vi "0254-initialization-reference.vi"(11 "0254-VISA":refnum<visa-resource-name>) -> (0 "error out":errorcluster, 2 "Executing Cmd":string, 3 "Execuiting Result":string)   [LabVIEW 2015]
uses:
  <vilib>/Instr/_visa.llb/VISA Configure Serial Port (Instr).vi
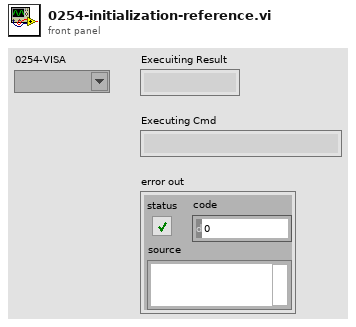
[diagram p1: front panel]
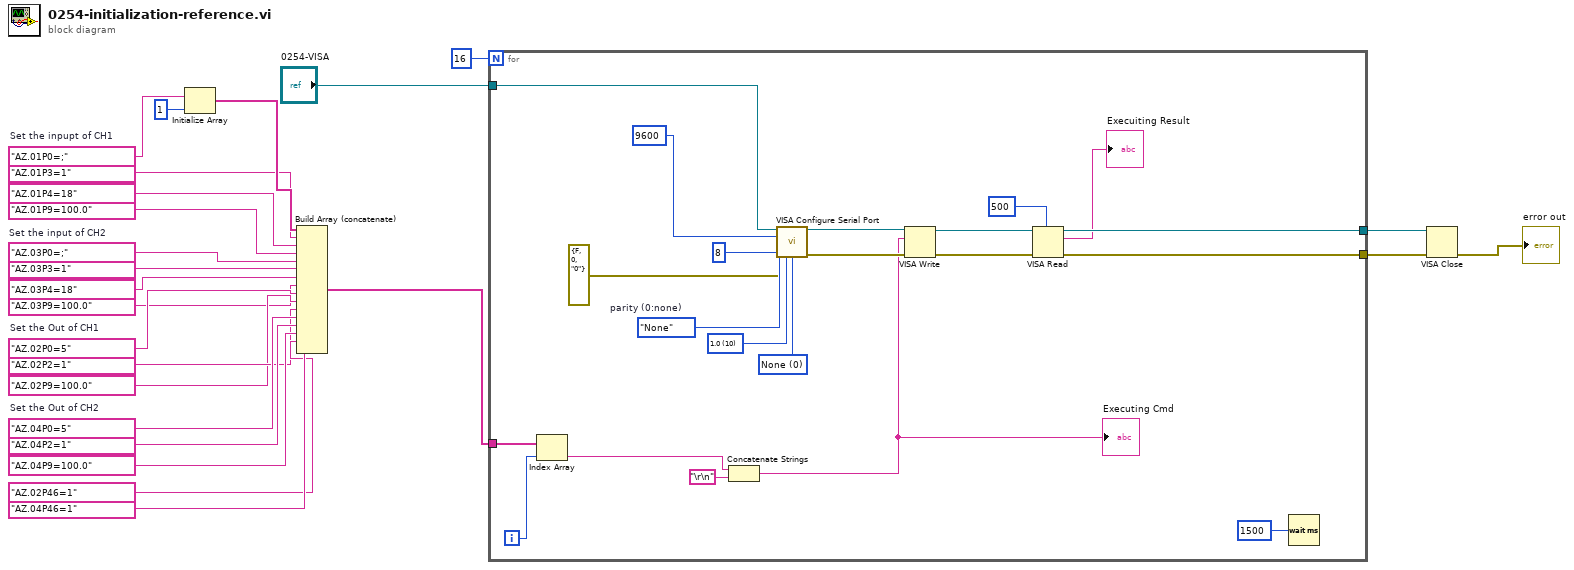
[diagram p0: block diagram]
diagram:
  w11 = "AZ.04P0=5"  # Set the Out of CH2
  w8 = "AZ.02P0=5"  # Set the Out of CH1
  w4 = "AZ.03P0=;"  # Set the input of CH2
  w18 = "AZ.01P0=;"  # Set the inpupt of CH1
  n1 = Initialize Array(w18, 1 ("dimension size")) -> (w20:string[])
  n2 = Build Array (concatenate)(w20, "AZ.01P3=1", "AZ.01P4=18", "AZ.01P9=100.0", w4, "AZ.03P3=1", "AZ.03P4=18", "AZ.03P9=100.0", w8, "AZ.02P9=100.0", "AZ.02P2=1", w11, "AZ.04P2=1", "AZ.04P9=100.0", "AZ.02P46=1", "AZ.04P46=1") -> (w21:string[])
  n3 = for {
    N: 16 -> [_]
    tunnel: [w29] -> w15
    tunnel: [w28] -> w16
    tunnel: "0254-VISA" -> [w27]
    tunnel: w21 -> [w26]
    i -> [w32]
    w37 = u16 0 items=["None", "XON/XOFF", "RTS/CTS", "XON/XOFF & RTS/CTS", "DTR/DSR", "XON/XOFF & DTR/DSR"] ("flow control (0:none)")
    w38 = u16 10 items=["1.0"=10, "1.5"=15, "2.0"=20] ("stop bits (10: 1 bit)")
    w40 = enum16{"None", "Odd", "Even", "Mark", "Space"}."None"  # parity (0:none)
    n4 = Index Array(array=w26, index=w32) -> (element=w31:string)
    n5 = Concatenate Strings(w31, "\r\n") -> (w33:string)
    "Executing Cmd" <- w33
    n6 = call-poly "VISA Configure Serial Port"("VISA resource name"=w27, "baud rate (9600)"=u32 9600, "data bits (8)"=u16 8, "parity (0:none)"=w40, "error in (no error)"=errorcluster {"status"=FALSE, "code"=0, "source"="0"}, "stop bits (10: 1 bit)"=w38, "flow control (0:none)"=w37) -> ("VISA resource name out"=w39:refnum<visa-resource-name>, "error out"=w36:errorcluster)  [unwired: 7 in]
    n7 = VISA Write(VISA resource name=w39, write buffer=w33, error in (no error)=w36) -> (VISA resource name out=w45:refnum<visa-resource-name>, error out=w43:errorcluster)  [unwired: 1 out]
    n8 = VISA Read(VISA resource name=w45, byte count=u32 500, error in (no error)=w43) -> (VISA resource name out=w28:refnum<visa-resource-name>, read buffer=→"Execuiting Result":string, error out=w29:errorcluster)  [unwired: 1 out]
    n9 = Wait (ms)(milliseconds to wait=u32 1500) -> ()  [unwired: 1 out]
  }
  n10 = VISA Close(VISA resource name=w16, error in (no error)=w15) -> (error out=→"error out":errorcluster)
